vi "P&Ts_Extract names from cluster control.vi"(8 "error in (no error)":errorcluster, 11 "Cluster 2":refnum<vi>) -> (0 "error out":errorcluster, 3 "Array":string[](array[string]))   [LabVIEW 2016]
uses:
  DAQLoop_Typedef.ctl
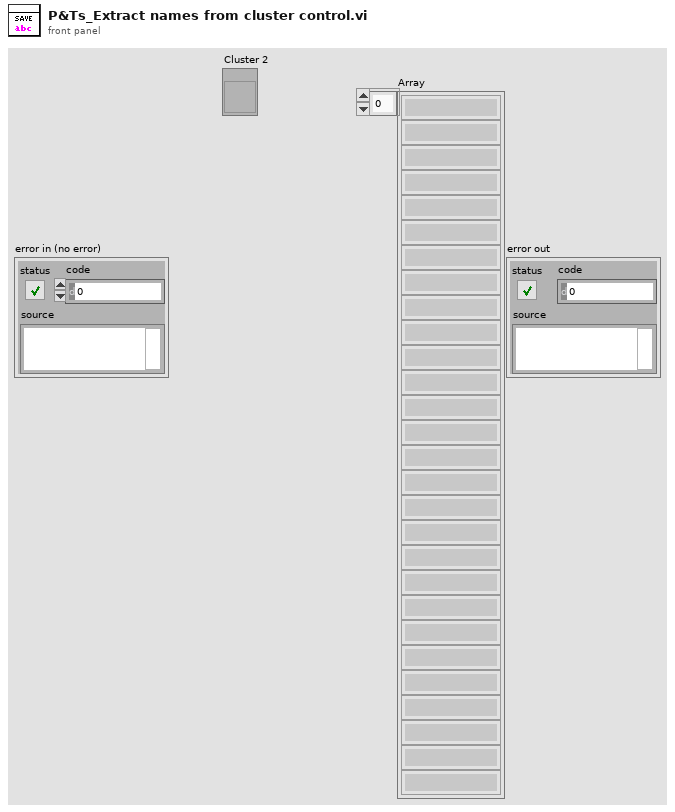
[diagram p1: front panel]
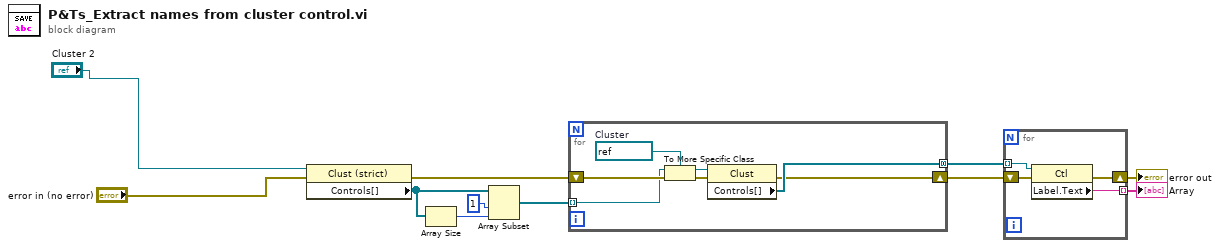
[diagram p0: block diagram]
diagram:
  n1 = property class="Clust (strict)"(reference="Cluster 2", error in="error in (no error)") -> (error out=w8:errorcluster, "Controls[]"=w6:refnum<vi>[])  [unwired: 1 out]
  n2 = Array Size(array=w6) -> (size(s)=w5:i32)
  n3 = Array Subset(array=w6, index=1, length=w5) -> (w3:refnum<vi>[])
  n4 = for {
    tunnel: w3 -> [w16] mode=indexing
    shift-right: [w12] -> w11
    shift-left: w8 -> [w18]
    tunnel: [w13] -> w10 mode=concatenating
    w17 = refnum<vi> refnum  # Cluster
    n5 = To More Specific Class(target class=w17, reference=w16, error in=w18) -> (specific class reference=w15:refnum<vi>, error out=w14:errorcluster)
    n6 = property class="Clust"(reference=w15, error in=w14) -> (error out=w12:errorcluster, "Controls[]"=w13:refnum<vi>[])  [unwired: 1 out]
  }
  n7 = for {
    shift-right: [w19] -> w2
    shift-left: w11 -> [w22]
    tunnel: w10 -> [w21] mode=indexing
    tunnel: [w20] -> w7 mode=indexing
    n8 = property class="Ctl"(reference=w21, error in=w22) -> (error out=w19:errorcluster, "Label.Text"=w20:string)  [unwired: 1 out]
  }
  "Array" <- w7
  "error out" <- w2
